vi "DBL Array To Mono-Item Text.vi"(10 "DBL Array":dbl[](array[numeric])) -> (2 "Mono-Item Text":string[](array[string]))   [LabVIEW 2024]
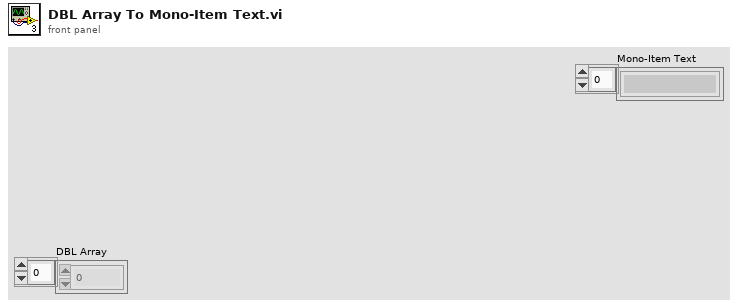
[diagram p1: front panel]
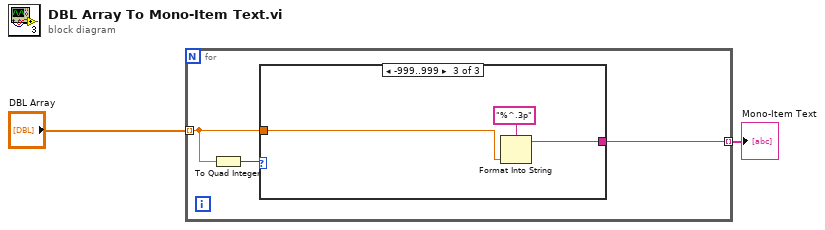
[diagram p0: block diagram]
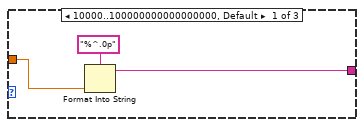
[diagram p2: hidden frame]
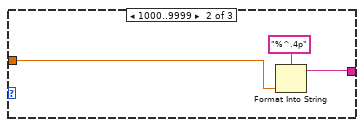
[diagram p3: hidden frame]
diagram:
  n1 = for {
    tunnel: "DBL Array" -> [w5] mode=indexing
    tunnel: [w3] -> w1 mode=indexing
    n2 = To Quad Integer(1:w5) -> (0:w4:i64)
    n3 = case shown="-999..999" w4 {
      tunnel: [w6 w10 w13] -> w3
      tunnel: w5 -> [w7 w9 w12]
      frame 10000..100000000000000000, Default {
        n4 = Format Into String(format string="%^.0p", w7) -> (resulting string=w6:string)  [unwired: 2 in, 1 out]
      }
      frame 1000..9999 {
        n5 = Format Into String(format string="%^.4p", w9) -> (resulting string=w10:string)  [unwired: 2 in, 1 out]
      }
      frame -999..999 {
        n6 = Format Into String(format string="%^.3p", w12) -> (resulting string=w13:string)  [unwired: 2 in, 1 out]
      }
    }
  }
  "Mono-Item Text" <- w1
